vi "Read Parameter Definition.vi"(8 "error in":errorcluster, 11 "parameter in":T3 format="%.0x") -> (0 "error out":errorcluster, 2 "parameter definition":T2, 3 "parameter out":T3 format="%.0x")   [LabVIEW 2020, in "Ballard MIL-STD-1553 Scripting.lvlib"]
uses:
  Ballard MIL-STD-1553 Scripting.lvlib
  <vilib>/NI VeriStand/Custom Device API/Custom Device Item Ref.ctl
  Shared/Parameter Definition.ctl
  Constants.vi
  <vilib>/NI VeriStand/Custom Device API/Get Item Property (String).vi
  <vilib>/NI VeriStand/Custom Device API/Get Item Property (Double).vi
  <vilib>/NI VeriStand/Custom Device API/Get Item Property (I32).vi
  <vilib>/NI VeriStand/Custom Device API/Get Item Property (U16).vi
  <vilib>/NI VeriStand/Custom Device API/Get Item Property (Boolean).vi
  <vilib>/NI VeriStand/Custom Device API/Custom Device API.lvlib
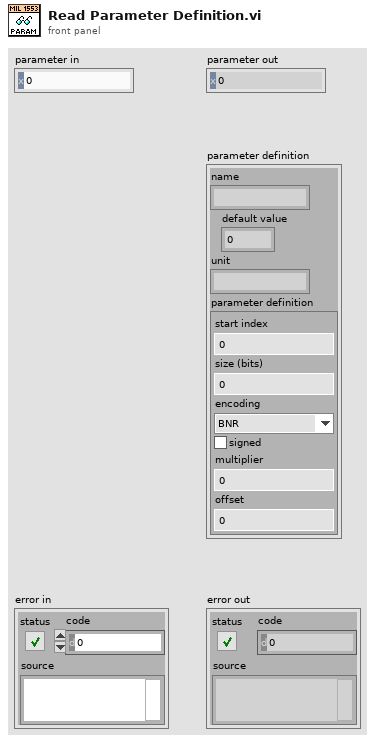
[diagram p1: front panel]
types:
  T1 = typedef "Parameter Definition.ctl" = cluster{"start index":i32, "size (bits)":i32, "encoding":enum16{"BNR", "BCD", "Discrete"}, "signed":bool, "multiplier":dbl, "offset":dbl}
  T2 = cluster{"name":string, "default value":dbl, "unit":string, "parameter definition":T1}
  T3 = typedef "Custom Device API.lvlib/Custom Device Item Ref.ctl" = u64
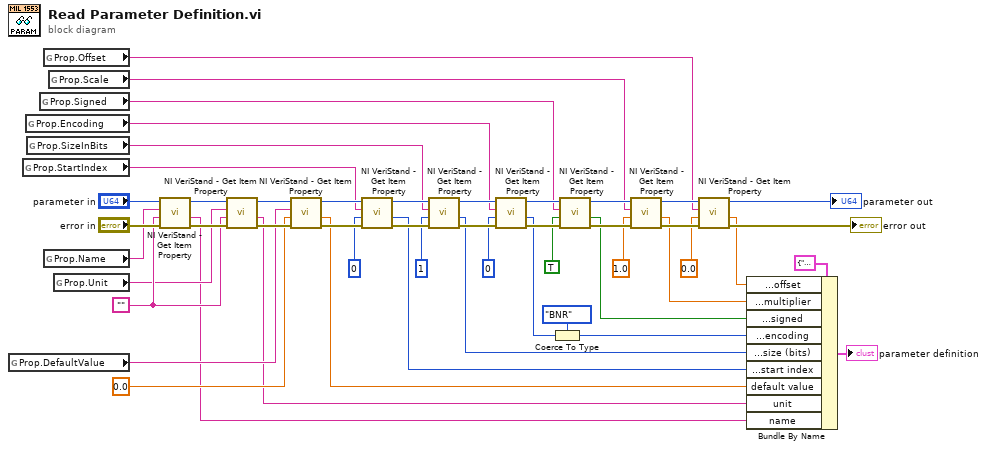
[diagram p0: block diagram]
diagram:
  w5 = "" ("name")
  n1 = global read "Constants.vi" "Prop.DefaultValue"() -> (w8:string)
  n2 = global read "Constants.vi" "Prop.StartIndex"() -> (w21:string)
  n3 = global read "Constants.vi" "Prop.Encoding"() -> (w23:string)
  n4 = global read "Constants.vi" "Prop.SizeInBits"() -> (w22:string)
  n5 = global read "Constants.vi" "Prop.Signed"() -> (w24:string)
  n6 = global read "Constants.vi" "Prop.Offset"() -> (w26:string)
  n7 = global read "Constants.vi" "Prop.Name"() -> (w6:string)
  n8 = global read "Constants.vi" "Prop.Scale"() -> (w25:string)
  n9 = global read "Constants.vi" "Prop.Unit"() -> (w4:string)
  n10 = call-poly <vilib>:"NI VeriStand - Get Item Property.vi"("error in (no error)"="error in", "Default Value"=w5, "Property Name"=w6, "Item Ref in"="parameter in") -> ("error out"=w45:errorcluster, "Value"=w1:string, "Item Ref out"=w46:T3)  [unwired: 4 in, 1 out]
  n11 = call-poly <vilib>:"NI VeriStand - Get Item Property.vi"("error in (no error)"=w45, "Default Value"=w5, "Property Name"=w4, "Item Ref in"=w46) -> ("error out"=w43:errorcluster, "Value"=w2:string, "Item Ref out"=w44:T3)  [unwired: 4 in, 1 out]
  n12 = call-poly <vilib>:"NI VeriStand - Get Item Property.vi"("error in (no error)"=w43, "Default Value"=0.0, "Property Name"=w8, "Item Ref in"=w44) -> ("error out"=w41:errorcluster, "Value"=w3:dbl, "Item Ref out"=w42:T3)  [unwired: 4 in, 1 out]
  n13 = call-poly <vilib>:"NI VeriStand - Get Item Property.vi"("error in (no error)"=w41, "Default Value"=0, "Property Name"=w21, "Item Ref in"=w42) -> ("error out"=w39:errorcluster, "Value"=w9:i32, "Item Ref out"=w40:T3)  [unwired: 4 in, 1 out]
  n14 = call-poly <vilib>:"NI VeriStand - Get Item Property.vi"("error in (no error)"=w39, "Default Value"=1, "Property Name"=w22, "Item Ref in"=w40) -> ("error out"=w37:errorcluster, "Value"=w11:i32, "Item Ref out"=w38:T3)  [unwired: 4 in, 1 out]
  n15 = call-poly <vilib>:"NI VeriStand - Get Item Property.vi"("error in (no error)"=w37, "Default Value"=u16 0, "Property Name"=w23, "Item Ref in"=w38) -> ("error out"=w35:errorcluster, "Value"=w13:u16, "Item Ref out"=w36:T3)  [unwired: 4 in, 1 out]
  n16 = Coerce To Type(0:w13, 1:enum16{"BNR", "BCD", "Discrete"}."BNR" ("parameter definition.encoding")) -> (2:w49:enum16{"BNR", "BCD", "Discrete"})
  n17 = call-poly <vilib>:"NI VeriStand - Get Item Property.vi"("error in (no error)"=w35, "Default Value"=TRUE ("required (F)"), "Property Name"=w24, "Item Ref in"=w36) -> ("error out"=w33:errorcluster, "Value"=w15:bool, "Item Ref out"=w34:T3)  [unwired: 4 in, 1 out]
  n18 = call-poly <vilib>:"NI VeriStand - Get Item Property.vi"("error in (no error)"=w33, "Default Value"=1.0, "Property Name"=w25, "Item Ref in"=w34) -> ("error out"=w31:errorcluster, "Value"=w16:dbl, "Item Ref out"=w32:T3)  [unwired: 4 in, 1 out]
  n19 = call-poly <vilib>:"NI VeriStand - Get Item Property.vi"("error in (no error)"=w31, "Default Value"=0.0, "Property Name"=w26, "Item Ref in"=w32) -> ("error out"=→"error out":errorcluster, "Value"=w18:dbl, "Item Ref out"=→"parameter out":T3)  [unwired: 4 in, 1 out]
  n20 = Bundle By Name(cluster=T2 {"name"="", "default value"=1.0, "unit"="", "parameter definition"={"start index"=0, "size (bits)"=16, "encoding"=enum."BNR", "signed"=FALSE, "multiplier"=1.0, "offset"=0.0}} ("definition with default value"), "parameter definition.offset"=w18, "parameter definition.multiplier"=w16, "parameter definition.signed"=w15, "parameter definition.encoding"=w49, "parameter definition.size (bits)"=w11, "parameter definition.start index"=w9, "default value"=w3, "unit"=w2, "name"=w1) -> (→"parameter definition":T2)
